vi "Main.vi"() -> ()   [LabVIEW 2020, in "WebServiceImporter.lvlib" / "Main Panel.lvlib" / "Progress.lvlib"]
uses:
  <vilib>/Platform/WebService/Main Panel/Pages/Progress/Progress.lvlib
  <vilib>/Platform/WebService/Main Panel/Pages/Progress/Events/Events.lvlib
panel:
  in  "Panel":enum32{"Interface Frame", "Hidden Controls"}(tab)
  out "Progress:":dbl(slide)=1.0 caption="Progress" scale=0.0..1.0
  # "Importing Web Service"
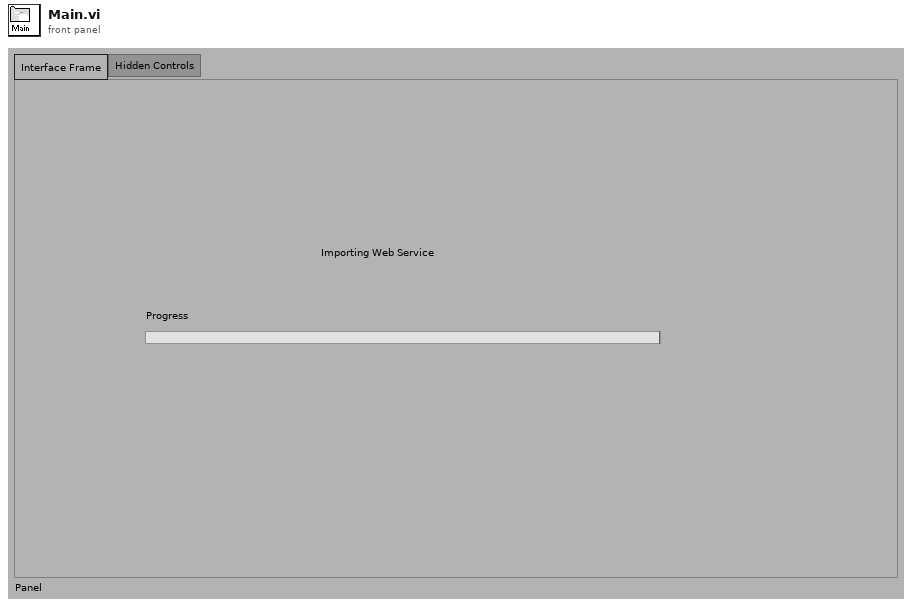
[diagram p1: front panel]
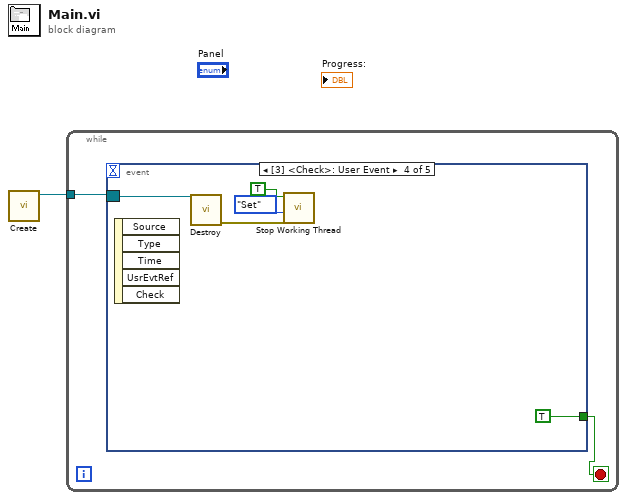
[diagram p0: block diagram]
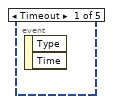
[diagram p2: hidden frame]
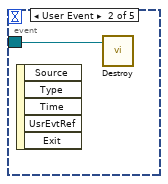
[diagram p3: hidden frame]
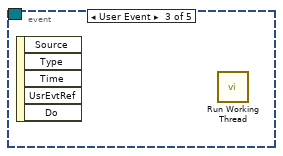
[diagram p4: hidden frame]
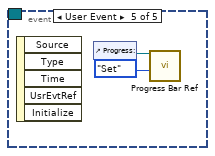
[diagram p5: hidden frame]
diagram:
  n1 = call <vilib>:"Create.vi"() -> ("Event Registration Refnum"=w1:refnum<event-registration>)  [unwired: 10 in, 1 out]
  n2 = while {
    tunnel: w1 -> [w3]
    stop <- w2 stop-if-true
    n3 = event shown="[3] <Check>: User Event" {
      selector: w3 -> [_ w4 _ w5 _]
      dyn-events: _ -> [_ _ _ _ _]
      timeout: _ -> [_ _ _ _ _]
      tunnel: [_ _ _ TRUE _] -> w2
      event Timeout {
        n4 = event-data() -> ()  [unwired: 1 in, 2 out]
      }
      event User Event {
        n5 = event-data() -> ()  [unwired: 1 in, 5 out]
        n6 = call <vilib>:"Destroy.vi"("Event Registration Refnum"=w4) -> ()  [unwired: 10 in, 1 out]
      }
      event User Event {
        n7 = event-data() -> ()  [unwired: 1 in, 5 out]
        n8 = call <vilib>:"Run Working Thread.vi"() -> ()  [unwired: 11 in, 1 out]
      }
      event User Event {
        n9 = event-data() -> ()  [unwired: 1 in, 5 out]
        n10 = call <vilib>:"Destroy.vi"("Event Registration Refnum"=w5) -> ("error out"=w6:errorcluster)  [unwired: 10 in]
        n11 = call <vilib>:"Stop Working Thread.vi"("error in (no error)"=w6, "Operation"=enum16{"Get", "Set"}."Set", "Stop the working thread"=TRUE) -> ()  [unwired: 7 in, 2 out]
      }
      event User Event {
        n12 = event-data() -> ()  [unwired: 1 in, 5 out]
        n13 = control-ref of="Progress:"() -> (w11:refnum<vi>)
        n14 = call <vilib>:"Progress Bar Ref.vi"("Operation"=enum16{"Get", "Set"}."Set", "Progress"=w11) -> ()  [unwired: 8 in, 2 out]
      }
    }
  }
